vi "Distributor - SET - Triggered Events & Data.vi"(8 "error in (no error)":errorcluster, 9 "Data":string, 10 "Events":T1, 11 "Parent_Class in":refnum<class "Message_Distributor_Class.lvclass">) -> (0 "error out":errorcluster, 3 "Parent_Class out":refnum<class "Message_Distributor_Class.lvclass">)   [LabVIEW 2023, in "Actor_Message_Distributor.lvlib" / "Message_Distributor_Class.lvclass"]
uses:
  Message_Distributor_Class.lvclass
  Usr Ev/Distributor - Ctrl - Enum - Events.ctl
  Message_Distributor_Class.lvclass/Message_Distributor_Class.ctl
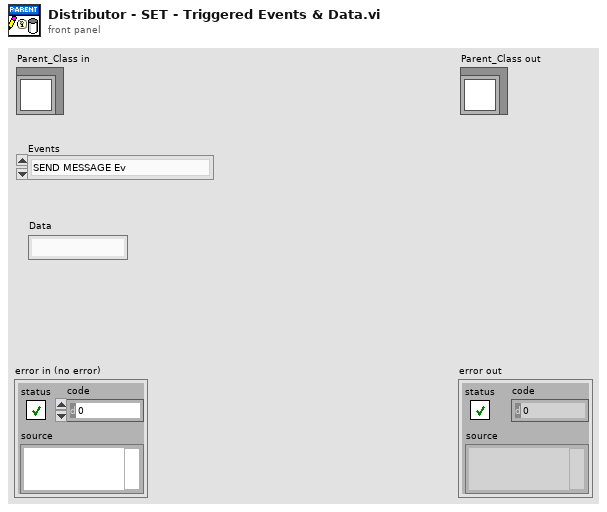
[diagram p1: front panel]
types:
  T1 = typedef "Actor_Message_Distributor.lvlib/Message_Distributor_Class.lvclass/Distributor - Ctrl - Enum - Events.ctl" = enum16{"SEND MESSAGE Ev", "STOP_ACTOR Ev", "INIT_ACTOR Ev", "START Ev", "STOP Ev", "GET Ev", "SET Ev", "ERROR_HANDLER Ev", "RESET Ev", "DISPATCH MESSAGE 2 CHILDS Ev", "ECU RESET Ev"}
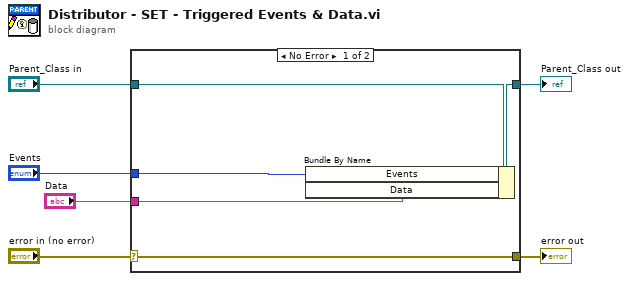
[diagram p0: block diagram]
diagram:
  n1 = case shown="No Error" "error in (no error)" {
    selector: "error in (no error)" -> [w11 w12]
    tunnel: [w11 w12] -> w5
    tunnel: [w9 w13] -> w3
    tunnel: "Parent_Class in" -> [w10 w13]
    tunnel: "Events" -> [w8 _]
    tunnel: "Data" -> [w7 _]
    frame No Error {
      n2 = Bundle By Name(cluster=w10, "Events"=w8, "Data"=w7) -> (w9:refnum<class "Message_Distributor_Class.lvclass">)
    }
    frame Error {
    }
  }
  "error out" <- w5
  "Parent_Class out" <- w3
